vi "Check Controls are Error Cluster.vi"(11 "Controls[]":refnum<vi>[](array[refnum])) -> (3 "Error Cluster":bool)   [LabVIEW 2023, in "VIDoc Parsing.lvlib"]
uses:
  VIDoc Parsing.lvlib
  <vilib>/numeric/LVNumericRepresentation.ctl
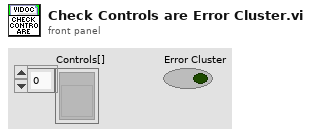
[diagram p1: front panel]
types:
  T1 = typedef "LVNumericRepresentation.ctl" = enum32{"Extended Precision", "Double Precision", "Single Precision", "Long", "Word", "Byte", "Unsigned Long", "Unsigned Word", "Unsigned Byte", "Complex Extended", "Complex Double", "Complex Single", "Quad", "Unsigned Quad", "Fixed-Point"}
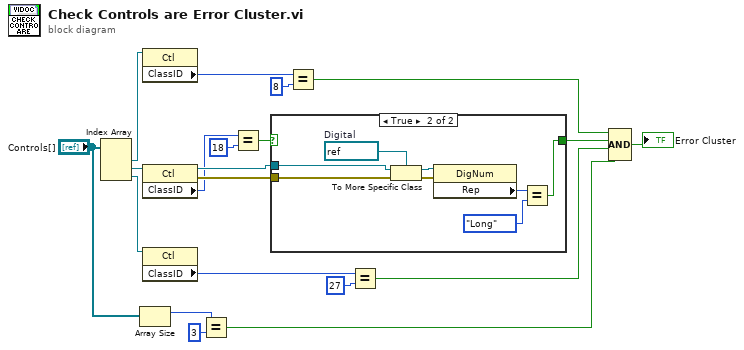
[diagram p0: block diagram]
diagram:
  n1 = Index Array(array="Controls[]") -> (element #1=w20:refnum<vi>, element #2=w19:refnum<vi>, element #3=w18:refnum<vi>)  [unwired: 3 in]
  n2 = Array Size(array="Controls[]") -> (size(s)=w3:i32)
  n3 = property class="Ctl"(reference=w20) -> ("ClassID"=w15:u32)  [unwired: 1 in, 2 out]
  n4 = property class="Ctl"(reference=w19) -> (reference out=w17:refnum<vi>, error out=w16:errorcluster, "ClassID"=w11:u32)  [unwired: 1 in]
  n5 = property class="Ctl"(reference=w18) -> ("ClassID"=w12:u32)  [unwired: 1 in, 2 out]
  n6 = Equal?(x=w3, y=3) -> (x = y?=w1:bool)
  n7 = Equal?(x=w11, y=u32 18) -> (x = y?=w9:bool)
  n8 = case shown="True" w9 {
    selector: w9 -> [w21 _]
    tunnel: w17 -> [_ w29]
    tunnel: w16 -> [_ w28]
    tunnel: [w21 w22] -> w8
    frame False {
    }
    frame True {
      w25 = refnum<vi> refnum  # Digital
      n9 = To More Specific Class(target class=w25, reference=w29, error in=w28) -> (specific class reference=w27:refnum<vi>, error out=w26:errorcluster)
      n10 = property class="DigNum"(reference=w27, error in=w26) -> ("Rep"=w24:T1)  [unwired: 2 out]
      n11 = Equal?(x=w24, y=LVNumericRepresentation."Long" ("Representation 2")) -> (x = y?=w22:bool)
    }
  }
  n12 = Equal?(x=w15, y=u32 8) -> (x = y?=w7:bool)
  n13 = Equal?(x=w12, y=u32 27) -> (x = y?=w6:bool)
  n14 = Compound Arithmetic op=AND(w7, w8, w6, w1) -> (→"Error Cluster":bool)
